vi "LOC subGetAllControlsInVI.vi"(4 "error in (no error)":errorcluster, 6 "IgnoreCtrlsWithLeading \"_\"":bool=TRUE, 7 "VIRefnum":refnum<vi>) -> (0 "error out":errorcluster, 2 "ControlLabels":string[](array[string]), 3 "ControlRefnums":refnum<vi>[](array[refnum]))   [LabVIEW 2020, in "Localization_Tools.lvlib"]
uses:
  Localization_Tools.lvlib
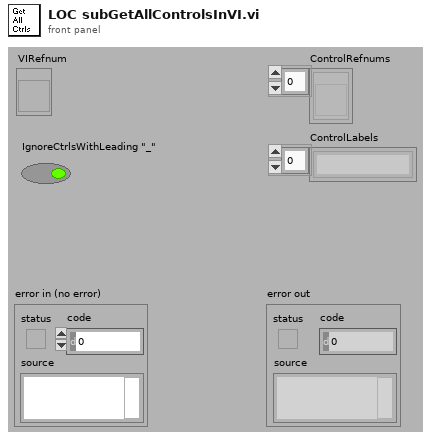
[diagram p1: front panel]
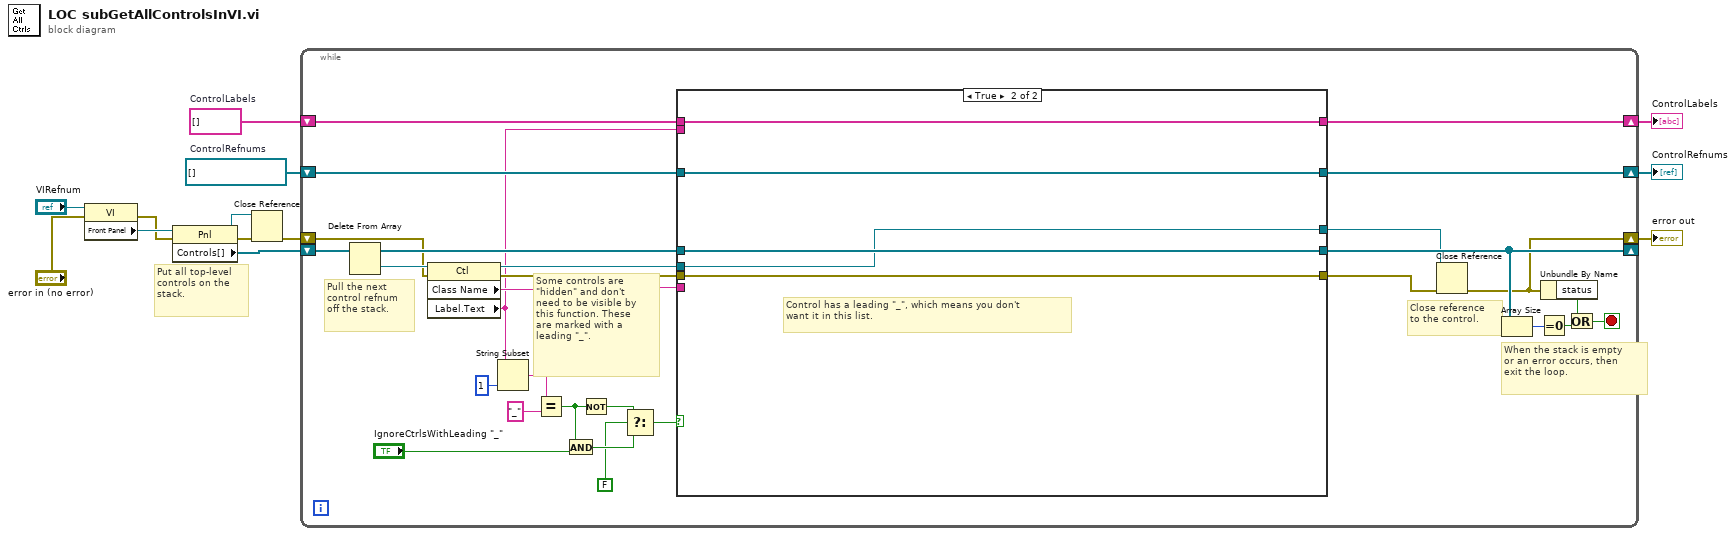
[diagram p0: block diagram]
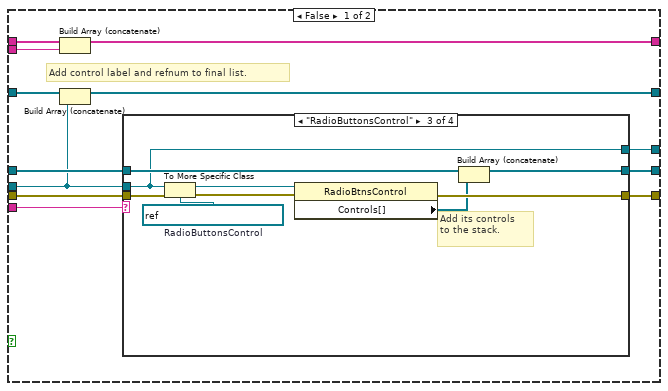
[diagram p2: hidden frame]
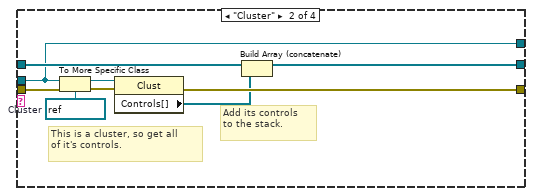
[diagram p4: hidden frame]
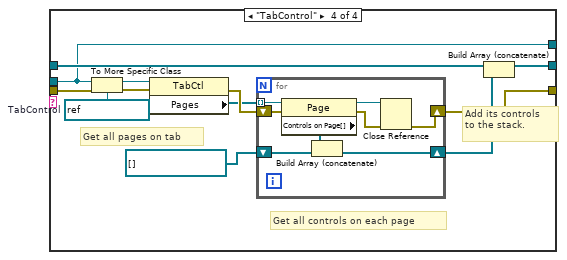
[diagram p5: hidden frame]
diagram:
  w2 = string[] []  # ControlLabels
  w11 = refnum<vi>[] []  # ControlRefnums
  # "Put all top-level\ncontrols on the\nstack."
  n1 = property class="VI"(reference="VIRefnum", error in="error in (no error)") -> (error out=w7:errorcluster, "Front Panel"=w13:refnum<vi>)  [unwired: 1 out]
  n2 = property class="Pnl"(reference=w13, error in=w7) -> (reference out=w4:refnum<vi>, error out=w5:errorcluster, "Controls[]"=w12:refnum<vi>[])
  n3 = Close Reference(reference=w4, error in (no error)=w5) -> (error out=w3:errorcluster)
  n4 = while {
    shift-right: [w38] -> _
    shift-left: w12 -> [w42]
    shift-right: [w26] -> w9
    shift-left: w11 -> [w28]
    shift-right: [w30] -> w6
    shift-left: w3 -> [w36]
    shift-right: [w24] -> w1
    shift-left: w2 -> [w25]
    stop <- w32 stop-if-true
    # "Some controls are\n\"hidden\" and don't\nneed to be visible by\nthis function. These\nare marked with a\nleading \"_\"."
    # "Close reference\nto the control."
    # "When the stack is empty\nor an error occurs, then\nexit the loop."
    # "Pull the next\ncontrol refnum\noff the stack."
    n5 = Delete From Array(array=w42) -> (deleted portion=w41:refnum<vi>, array with subset deleted=w39:refnum<vi>[])  [unwired: 2 in]
    n6 = property class="Ctl"(reference=w41, error in=w36) -> (reference out=w27:refnum<vi>, error out=w35:errorcluster, "Class Name"=w40:string, "Label.Text"=w22:string)
    n7 = String Subset(string=w22, length (rest)=1 ("length (rest)")) -> (substring=w21:string)  [unwired: 1 in]
    n8 = Equal?(x=w21, y="_") -> (x = y?=w16:bool)
    n9 = And(x=w16, y="IgnoreCtrlsWithLeading \"_\"") -> (x .and. y?=w18:bool)
    n10 = Not(x=w16) -> (.not. x?=w15:bool)
    n11 = Select(t=w15, s=FALSE, f=w18) -> (s? t:f=w17:bool)
    n12 = case shown="True" w17 {
      tunnel: w40 -> [w54 _]
      tunnel: w39 -> [w53 w98]
      tunnel: [w52 w98] -> w38
      tunnel: w35 -> [w51 w96]
      tunnel: [w50 w96] -> w31
      tunnel: [w49 w97] -> w29
      tunnel: w28 -> [w48 w99]
      tunnel: w27 -> [w47 w97]
      tunnel: [w46 w99] -> w26
      tunnel: w25 -> [w45 w100]
      tunnel: [w44 w100] -> w24
      tunnel: w22 -> [w43 _]
      frame False {
        # "Add control label and refnum to final list."
        n13 = Build Array (concatenate)(w45, w43) -> (w44:string[])
        n14 = Build Array (concatenate)(w48, w47) -> (w46:refnum<vi>[])
        n15 = case shown="\"RadioButtonsControl\"" w54 {
          tunnel: w47 -> [w55 w58 w67 w81]
          tunnel: w53 -> [w57 w60 w69 w83]
          tunnel: [w57 w59 w68 w82] -> w52
          tunnel: w51 -> [w56 w63 w72 w84]
          tunnel: [w56 w62 w71 w76] -> w50
          tunnel: [w55 w58 w67 w81] -> w49
          frame Default {
            # "This is a singular element."
          }
          frame "Cluster" {
            w66 = refnum<vi> refnum  # Cluster
            # "Add its controls\nto the stack."
            # "This is a cluster, so get all\nof it's controls."
            n16 = To More Specific Class(target class=w66, reference=w58, error in=w63) -> (specific class reference=w65:refnum<vi>, error out=w64:errorcluster)
            n17 = property class="Clust"(reference=w65, error in=w64) -> (error out=w62:errorcluster, "Controls[]"=w61:refnum<vi>[])  [unwired: 1 out]
            n18 = Build Array (concatenate)(w60, w61) -> (w59:refnum<vi>[])
          }
          frame "RadioButtonsControl" {
            w75 = refnum<vi> refnum  # RadioButtonsControl
            # "Add its controls\nto the stack."
            n19 = To More Specific Class(target class=w75, reference=w67, error in=w72) -> (specific class reference=w74:refnum<vi>, error out=w73:errorcluster)
            n20 = property class="RadioBtnsControl"(reference=w74, error in=w73) -> (error out=w71:errorcluster, "Controls[]"=w70:refnum<vi>[])  [unwired: 1 out]
            n21 = Build Array (concatenate)(w69, w70) -> (w68:refnum<vi>[])
          }
          frame "TabControl" {
            w87 = refnum<vi> refnum  # TabControl
            # "Get all controls on each page"
            # "Add its controls\nto the stack."
            # "Get all pages on tab"
            n22 = To More Specific Class(target class=w87, reference=w81, error in=w84) -> (specific class reference=w86:refnum<vi>, error out=w85:errorcluster)
            n23 = property class="TabCtl"(reference=w86, error in=w85) -> (error out=w80:errorcluster, "Pages"=w79:refnum<vi>[])  [unwired: 1 out]
            n24 = for {
              tunnel: w79 -> [w95] mode=indexing
              shift-right: [w88] -> w76
              shift-left: w80 -> [w94]
              shift-right: [w91] -> w77
              shift-left: refnum<vi>[] [] ("Controls on Page[]") -> [w92]
              n25 = property class="Page"(reference=w95, error in=w94) -> (reference out=w90:refnum<vi>, error out=w89:errorcluster, "Controls on Page[]"=w93:refnum<vi>[])
              n26 = Build Array (concatenate)(w93, w92) -> (w91:refnum<vi>[])
              n27 = Close Reference(reference=w90, error in (no error)=w89) -> (error out=w88:errorcluster)
            }
            n28 = Build Array (concatenate)(w83, w77) -> (w82:refnum<vi>[])
          }
        }
      }
      frame True {
        # "Control has a leading \"_\", which means you don't\nwant it in this list."
      }
    }
    n29 = Close Reference(reference=w29, error in (no error)=w31) -> (error out=w30:errorcluster)
    n30 = Array Size(array=w38) -> (size(s)=w37:i32)
    n31 = Equal To 0?(x=w37) -> (x = 0?=w33:bool)
    n32 = Unbundle By Name(w30) -> ("status"=w34:bool)
    n33 = Or(x=w34, y=w33) -> (x .or. y?=w32:bool)
  }
  "ControlRefnums" <- w9
  "error out" <- w6
  "ControlLabels" <- w1
